vi "PTSequencer.remove unused DIM subscriptions.vi"(0 "DIM subsriptions":string[](array[string]), 2 "Used subsriptions":string[](array[string])) -> (14 "DIM subsriptions out":string[](array[string]), 18 "msgs to remove":T1[](array[typedef]))   [LabVIEW 2014, in "PTSequencer.lvlib"]
uses:
  PTSequencer.lvlib
  CS_Core/BaseProcess/BaseProcess.event definition.ctl
  CS_Core/CAEObj/CAEObj.event definition.ctl
  CS_Core/BaseProcess/BaseProcess.descriptor string definition.ctl
  CS_Core/BaseProcess/BaseProcess.lvlib
  CS_Core/CAEObj/CAEObj.lvlib
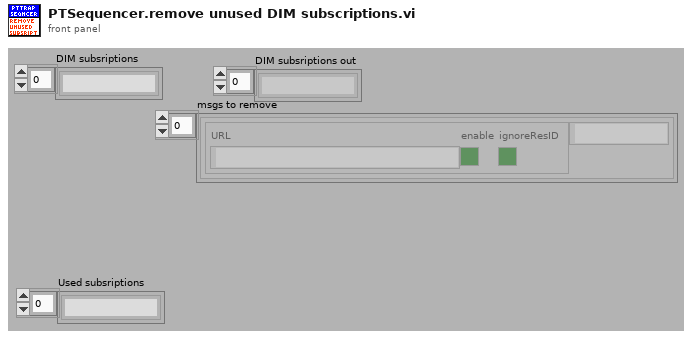
[diagram p1: front panel]
types:
  T1 = typedef "BaseProcess.lvlib/BaseProcess.event definition.ctl" = cluster{"CAEEvtDef":T2, "Data Descriptor":T3}
  T2 = typedef "CAEObj.lvlib/CAEObj.event definition.ctl" = cluster{"URL":string, "enable":bool, "ignoreResID":bool}
  T3 = typedef "BaseProcess.lvlib/BaseProcess.descriptor string definition.ctl" = string
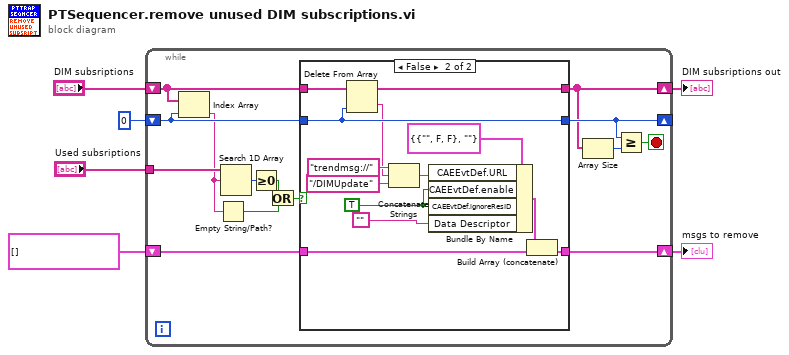
[diagram p0: block diagram]
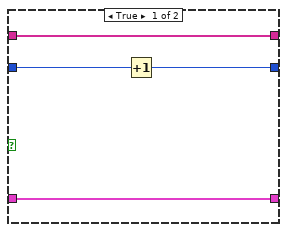
[diagram p2: hidden frame]
diagram:
  n1 = while {
    tunnel: "Used subsriptions" -> [w20]
    shift-right: [w13] -> w2
    shift-left: "DIM subsriptions" -> [w19]
    shift-right: [w14] -> _
    shift-left: 0 -> [w18]
    shift-right: [w16] -> w1
    shift-left: T1[] [] -> [w17]
    stop <- w12 stop-if-true
    n2 = Index Array(array=w19, index=w18) -> (element=w11:string)
    n3 = Empty String/Path?(string/path=w11) -> (empty?=w9:bool)
    n4 = Search 1D Array(1D array=w20, element=w11) -> (index of element=w10:i32)  [unwired: 1 in]
    n5 = Greater Or Equal To 0?(x=w10) -> (x >= 0?=w8:bool)
    n6 = Or(x=w8, y=w9) -> (x .or. y?=w7:bool)
    n7 = case shown="False" w7 {
      tunnel: w19 -> [w24 w37]
      tunnel: [w24 w36] -> w13
      tunnel: w18 -> [w23 w35]
      tunnel: [w22 w35] -> w14
      tunnel: w17 -> [w21 w28]
      tunnel: [w21 w27] -> w16
      frame True {
        n8 = Increment(x=w23) -> (x+1=w22:i32)
      }
      frame False {
        w30 = TRUE ("CAEEvtDef.ignoreResID")
        n9 = Delete From Array(array=w37, index=w35) -> (deleted portion=w25:string, array with subset deleted=w36:string[])  [unwired: 1 in]
        n10 = Concatenate Strings("trendmsg://", w25, "/DIMUpdate" ("string")) -> (w31:string)
        n11 = Bundle By Name(cluster=T1 {"CAEEvtDef"={"URL"="", "enable"=FALSE, "ignoreResID"=FALSE}, "Data Descriptor"=""} ("event definition"), "CAEEvtDef.URL"=w31, "CAEEvtDef.enable"=w30, "CAEEvtDef.ignoreResID"=w30, "Data Descriptor"="") -> (w26:T1)
        n12 = Build Array (concatenate)(w26, w28) -> (w27:T1[])
      }
    }
    n13 = Array Size(array=w13) -> (size(s)=w15:i32)
    n14 = Greater Or Equal?(x=w14, y=w15) -> (x >= y?=w12:bool)
  }
  "DIM subsriptions out" <- w2
  "msgs to remove" <- w1
